vi "ShowData.vi"(11 "data in":refnum<class "EventMessengerData.lvclass">) -> (0 "aborted?":bool, 1 "high priority?":bool, 2 "write count":u32, 3 "data out":refnum<class "EventMessengerData.lvclass">, 4 "last element?":bool)   [LabVIEW 2019, in "Cmd-Data Event Messenger.lvlib" / "EventMessengerData.lvclass"]
uses:
  EventMessengerData.lvclass
  EventMessengerData.lvclass/EventMessengerData.ctl
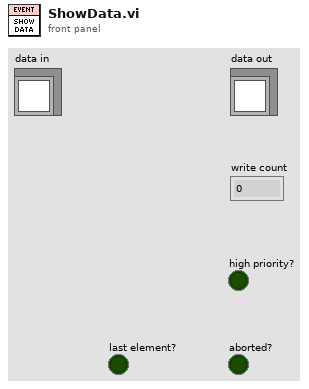
[diagram p1: front panel]
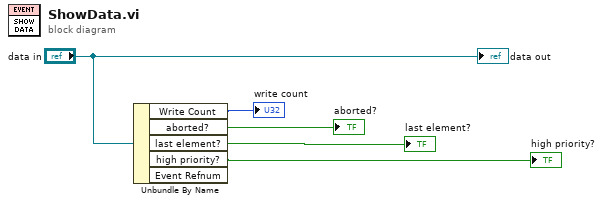
[diagram p0: block diagram]
diagram:
  n1 = Unbundle By Name("data in") -> ("Write Count"=→"write count":u32, "aborted?"=→"aborted?":bool, "last element?"=→"last element?":bool, "high priority?"=→"high priority?":bool)  [unwired: 1 out]
  "data out" <- "data in"
